vi "Main.vi"(11 "Module Admin":refnum<class "Delacor_lib_QMH_Module Admin.lvclass">) -> ()   [LabVIEW 2024, in "ProductControl.lvlib"]
doc: "This template is based off of the Queued Message Handler design pattern and the Queued Message Handler project template that ships with LabVIEW.\n\nThe main difference is that the queue is private to this module and communication between modules is performed via Broadcast and Request events.\n\nRequest events are wrapped in public API methods and are handled in the Event Handling Loop (EHL) of this VI. Any module can register for Broadcast events sent by this module. The EHL generates messages based on user interface actions.\n\nThe Message Handling Loop (MHL) processes messages generated by the EHL, or by other messages. The messages are string values, so new messages can be added easily to the Message Cases case structure in the MHL. Each message cluster can also provide an optional value for Message Data, which is a variant that can be converted to whatever message-specific data is required.\n_____\nBased on DQMH Dev Tools: Project Template 7.1.0.1503."
uses:
  ProductControl.lvlib
  <vilib>/Delacor/Delacor QMH/Libraries/Module Admin_class/Delacor_lib_QMH_Module Admin.lvclass
  Module Data--cluster.ctl
  <vilib>/Utility/miscctls.llb/LVFontTypeDef.ctl
  Stop Argument--cluster.ctl
  <vilib>/Delacor/Delacor QMH/Libraries/Message Queue_class/Delacor_lib_QMH_Message Queue.lvclass/Delacor_lib_QMH_Message Queue.ctl
  <vilib>/Delacor/Delacor QMH/Libraries/Module Admin_class/Delacor_lib_QMH_Module Admin.lvclass/Delacor_lib_QMH_Module Admin.ctl
  Draw FP in Subpanel Argument--cluster.ctl
  Remove From Subpanel Argument--cluster.ctl
  Cargar Invenario Argument--cluster.ctl
  <vilib>/Delacor/Delacor QMH/Libraries/Message Queue_class/Delacor_lib_QMH_Enqueue Message (Single).vi
  <vilib>/Delacor/Delacor QMH/Libraries/Module Admin_class/Delacor_lib_QMH_Get External Launch.vi
  <vilib>/Delacor/Delacor QMH/Libraries/Message Queue_class/Delacor_lib_QMH_Message Queue.lvclass
  <vilib>/PantherLAB/Message Module/Libraries/Message/PantherLAB_lib_Message.lvlib
  <vilib>/PantherLAB/Table Module/src/Libraries/Table/PantherLAB_lib_Table.lvlib
panel:
  out "error out":errorcluster
  out "Status":string
  in  "Comprar":bool
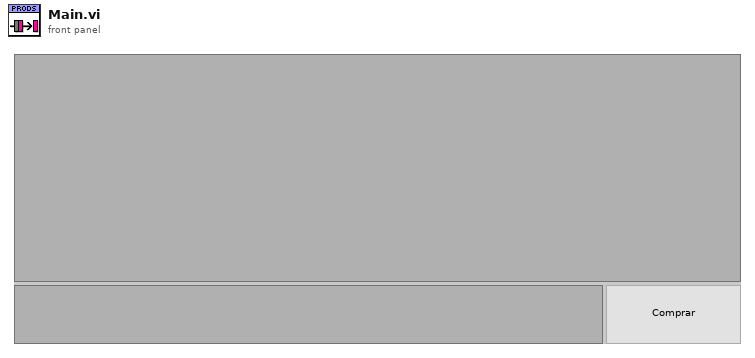
[diagram p1: front panel]
types:
  T1 = typedef "ProductControl.lvlib/Request Events--cluster.ctl" = cluster{"Stop Module":refnum<user-event>, "Show Panel":refnum<user-event>, "Hide Panel":refnum<user-event>, "Get Module Execution Status":refnum<user-event>, "Show Diagram":refnum<user-event>, "Draw FP in Subpanel":refnum<user-event>, "Remove From Subpanel":refnum<user-event>, "Private.Cargar Invenario":refnum<user-event>}
  T2 = typedef "PantherLAB_lib_Message.lvlib/Broadcast Events--cluster.ctl" = cluster{"Module Did Init":refnum<user-event>, "Status Updated":refnum<user-event>, "Error Reported":refnum<user-event>, "Module Did Stop":refnum<user-event>, "Update Module Execution Status":refnum<user-event>}
  T3 = typedef "PantherLAB_lib_Table.lvlib/Broadcast Events--cluster.ctl" = cluster{"Module Did Init":refnum<user-event>, "Status Updated":refnum<user-event>, "Error Reported":refnum<user-event>, "Module Did Stop":refnum<user-event>, "Update Module Execution Status":refnum<user-event>, "Selection Changed":refnum<user-event>}
  T4 = typedef "ProductControl.lvlib/Module Data--cluster.ctl" = cluster{"Status":string, "Sub Panel":refnum<vi>}
  T5 = typedef "LVFontTypeDef.ctl" = cluster{"Font Name":string, "Size":u16, "Bold":bool, "Italic":bool, "Underline":bool, "Strikeout":bool, "Color":u32}
  T6 = enum32{"invalid lock state", "Not Locked", "Locked (No Password)", "Password-protected"}
  T7 = typedef "ProductControl.lvlib/Stop Argument--cluster.ctl" = cluster{"Origin":string, "Exit via Stop Module Req?":bool, "Wait for Module to stop?":bool}
  T8 = typedef "ProductControl.lvlib/Draw FP in Subpanel Argument--cluster.ctl" = cluster{"Sub Panel":refnum<vi>}
  T9 = typedef "ProductControl.lvlib/Remove From Subpanel Argument--cluster.ctl" = cluster{"Boolean":bool}
  T10 = typedef "ProductControl.lvlib/Cargar Invenario Argument--cluster.ctl" = cluster{"Boolean":bool}
  T11 = enum32{"Invalid", "Standard", "Closed", "Hidden", "Minimized", "Maximized"}
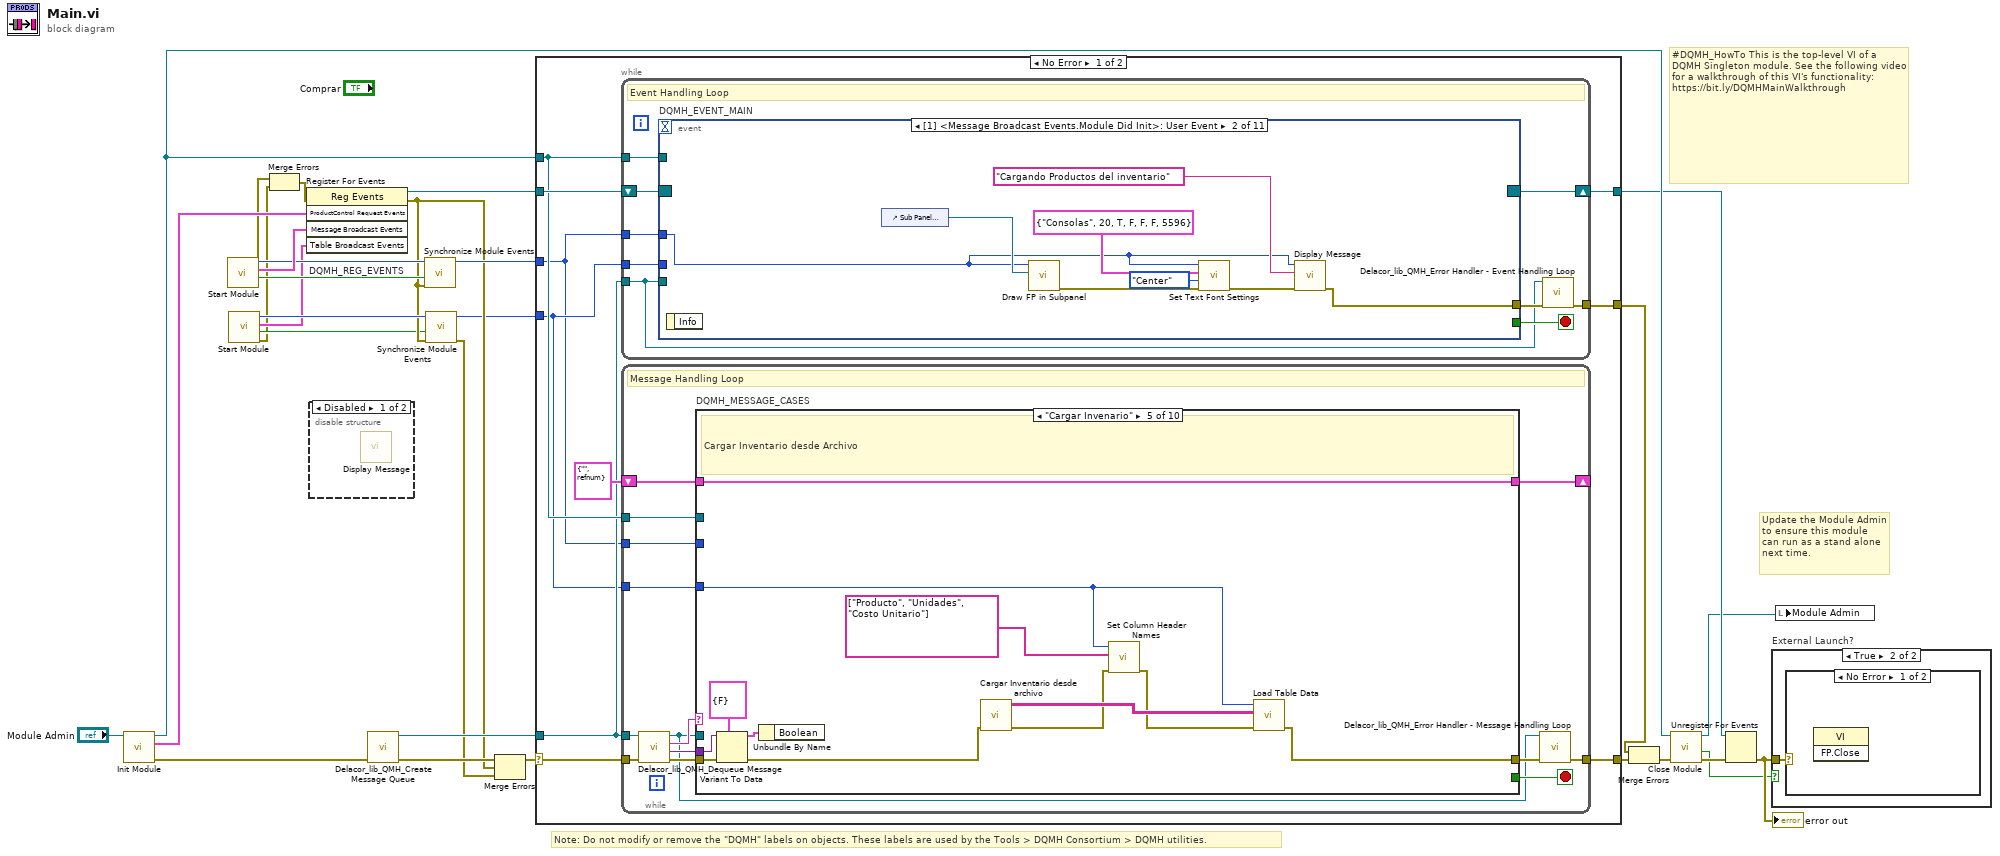
[diagram p0: block diagram]
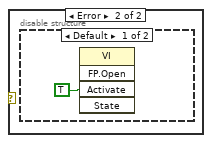
[diagram p4: hidden frame]
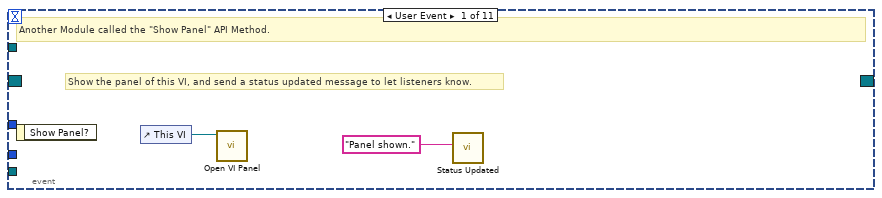
[diagram p6: hidden frame]
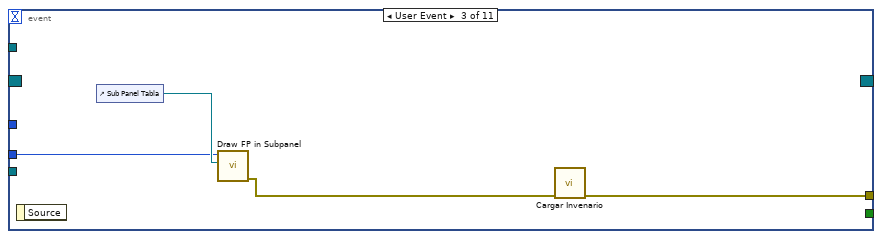
[diagram p7: hidden frame]
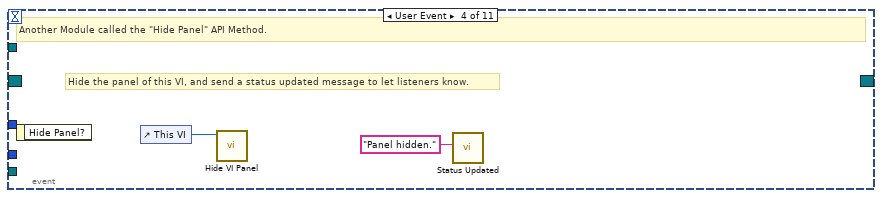
[diagram p8: hidden frame]
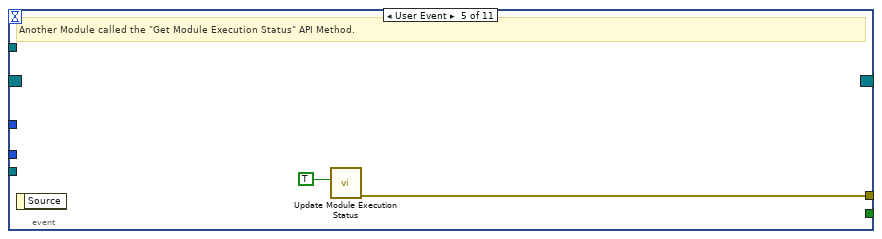
[diagram p9: hidden frame]
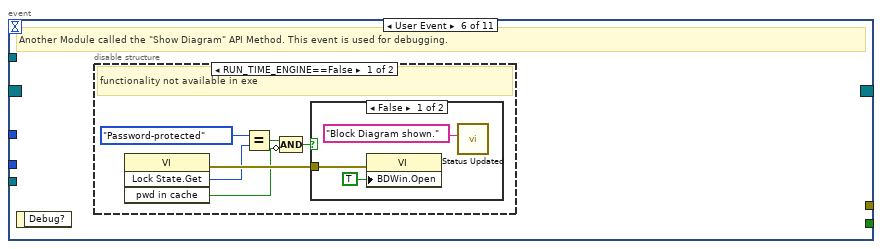
[diagram p10: hidden frame]
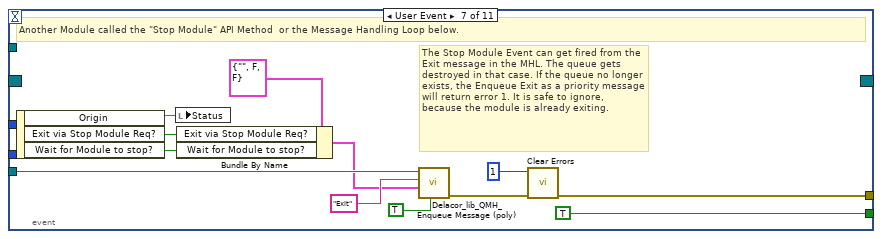
[diagram p13: hidden frame]
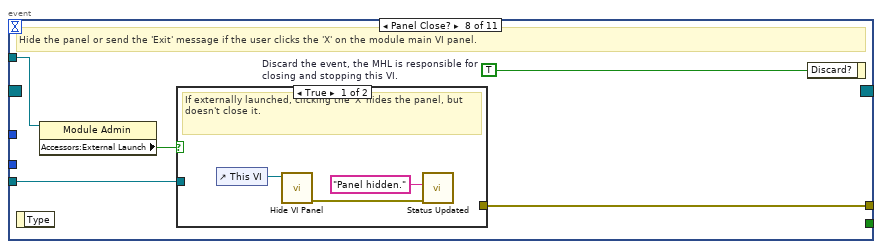
[diagram p14: hidden frame]
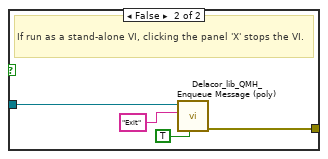
[diagram p15: hidden frame]
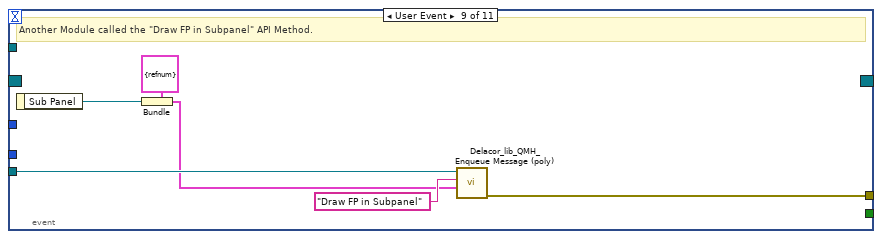
[diagram p16: hidden frame]
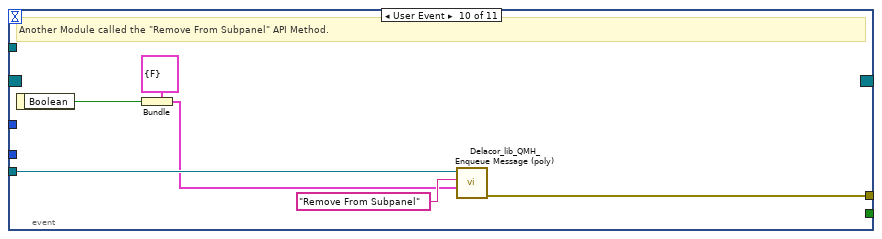
[diagram p17: hidden frame]
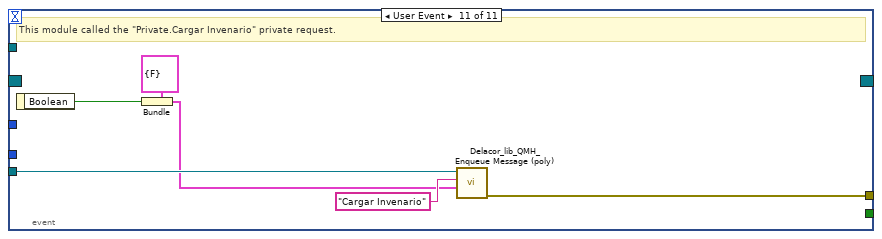
[diagram p18: hidden frame]
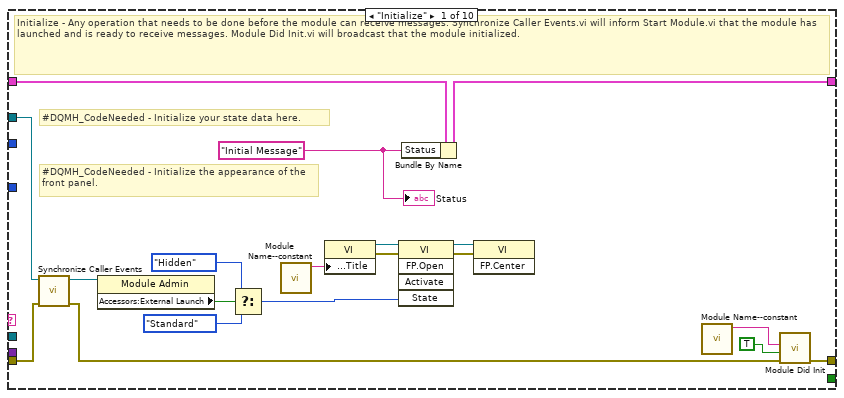
[diagram p19: hidden frame]
diagram:
  # "#DQMH_HowTo This is the top-level VI of a DQMH Singleton module. See the following video for a walkthrough of this VI's functionality: https://bit.ly/DQMHMainWalkthrough"
  # "Note: Do not modify or remove the \"DQMH\" labels on objects. These labels are used by the Tools > DQMH Consortium > DQMH utilities."
  # "Update the Module Admin to ensure this module can run as a stand alone next time."
  n1 = call "Init Module.vi"("Singleton Module Admin in"="Module Admin") -> ("error out"=w28:errorcluster, "ProductControl Request Events"=w18:T1, "Singleton Module Admin out"=w21:refnum<class "Delacor_lib_QMH_Module Admin.lvclass">)  [unwired: 8 in]
  n2 = call <vilib>:"Start Module.vi"() -> ("error out"=w9:errorcluster, "Wait for Event Sync?"=w12:bool, "Message Broadcast Events"=w11:T2, "Module ID"=w10:i32)  [unwired: 7 in, 1 out]
  n3 = call <vilib>:"Start Module.vi"() -> ("error out"=w2:errorcluster, "Wait for Event Sync?"=w4:bool, "Table Broadcast Events"=w5:T3, "Module ID"=w8:i32)  [unwired: 7 in, 1 out]
  n4 = Merge Errors(w9, w2) -> (w3:errorcluster)
  n5 = register-events "DQMH_REG_EVENTS"(error in=w3, w18, w11, w5) -> (reference out=w19:refnum<event-registration>, error out=w7:errorcluster)  [unwired: 1 in]
  n6 = disable-structure shown="Disabled" {
    frame Disabled {
      n7 = call <vilib>:"Display Message.vi"() -> ()  [unwired: 11 in, 1 out]
    }
    frame Enabled {
    }
  }
  n8 = call <vilib>:"Delacor_lib_QMH_Create Message Queue.vi"("error in"=w28) -> ("error out"=w23:errorcluster, "Message Queue"=w17:refnum<class "Delacor_lib_QMH_Message Queue.lvclass">)  [unwired: 9 in]
  n9 = call <vilib>:"Synchronize Module Events.vi"("error in"=w7, "Wait for Event Sync?"=w12, "Module ID in"=w10) -> ("Module ID out"=w13:i32)  [unwired: 7 in, 1 out]
  n10 = call <vilib>:"Synchronize Module Events.vi"("error in"=w7, "Wait for Event Sync?"=w4, "Module ID in"=w8) -> ("error out"=w6:errorcluster, "Module ID out"=w1:i32)  [unwired: 7 in]
  n11 = Merge Errors(w23, w7, w6) -> (w22:errorcluster)
  n12 = case shown="No Error" w22 {
    selector: w22 -> [w37 w262]
    tunnel: [w39 w261] -> w29
    tunnel: [w36 w260] -> w20
    tunnel: w19 -> [w34 w260]
    tunnel: w17 -> [w32 w256]
    tunnel: [w38 _] -> w26
    tunnel: w21 -> [w33 w257]
    tunnel: w13 -> [w30 w254]
    tunnel: w1 -> [w31 _]
    frame No Error {
      n13 = while {
        tunnel: w32 -> [w42]
        shift-right: [w45] -> w36
        shift-left: w34 -> [w46]
        tunnel: [w47] -> w38
        tunnel: w33 -> [w43]
        tunnel: w31 -> [w41]
        tunnel: w30 -> [w40]
        stop <- w44 stop-if-true
        # "Event Handling Loop"
        n14 = event "DQMH_EVENT_MAIN" shown="[1] <Message Broadcast Events.Module Did Init>: User Event" {
          selector: w46 -> [_ _ _ _ _ _ _ _ _ _ _]
          dyn-events: [_ _ _ _ _ _ _ _ _ _ _] -> w45
          timeout: _ -> [_ _ _ _ _ _ _ _ _ _ _]
          tunnel: [_ _ _ _ _ _ TRUE ("Discard?") _ _ _ _] -> w44
          tunnel: w42 -> [_ _ _ _ _ _ w83 w90 w104 w110 w117]
          tunnel: [_ w55 w60 _ w66 _ w86 w92 w105 w111 w112] -> w48
          tunnel: w43 -> [_ _ _ _ _ _ _ w89 _ _ _]
          tunnel: w41 -> [_ _ w59 _ _ _ _ _ _ _ _]
          tunnel: w40 -> [_ w51 _ _ _ _ _ _ _ _ _]
          event User Event {
            # "Show the panel of this VI, and send a status updated message to let listeners know."
            # "Another Module called the \"Show Panel\" API Method."
            n15 = event-data() -> ()  [unwired: 1 in, 1 out]
            n16 = control-ref of="This VI"() -> (w50:refnum<vi>)
            n17 = call "Open VI Panel.vi"("VI"=w50) -> ()  [unwired: 10 in, 1 out]
            n18 = call "Status Updated.vi"("Status"="Panel shown." ("format string")) -> ()  [unwired: 10 in, 1 out]
          }
          event User Event {
            n19 = event-data() -> ()  [unwired: 1 in, 1 out]
            n20 = control-ref of="Sub Panel Mensajes"() -> (w58:refnum<vi>)
            n21 = call <vilib>:"Draw FP in Subpanel.vi"("Sub Panel"=w58, "Module ID"=w51) -> ("error out"=w57:errorcluster)  [unwired: 9 in]
            n22 = call <vilib>:"Set Text Font Settings.vi"("error in"=w57, "Text.Justification"=enum16{"Left", "Center", "Right"}."Center", "Font"=T5 {"Font Name"="Consolas", "Size"=20, "Bold"=TRUE, "Italic"=FALSE, "Underline"=FALSE, "Strikeout"=FALSE, "Color"=5596}, "Module ID"=w51) -> ("error out"=w56:errorcluster)  [unwired: 7 in]
            n23 = call <vilib>:"Display Message.vi"("error in"=w56, "Message"="Cargando Productos del inventario", "Module ID"=w51) -> ("error out"=w55:errorcluster)  [unwired: 8 in]
          }
          event User Event {
            n24 = event-data() -> ()  [unwired: 1 in, 1 out]
            n25 = control-ref of="Sub Panel Tabla"() -> (w62:refnum<vi>)
            n26 = call <vilib>:"Draw FP in Subpanel.vi"("Sub Panel"=w62, "Module ID"=w59) -> ("error out"=w61:errorcluster)  [unwired: 9 in]
            n27 = call "Cargar Invenario.vi"("error in"=w61) -> ("error out"=w60:errorcluster)  [unwired: 10 in]
          }
          event User Event {
            # "Hide the panel of this VI, and send a status updated message to let listeners know."
            # "Another Module called the \"Hide Panel\" API Method."
            n28 = event-data() -> ()  [unwired: 1 in, 1 out]
            n29 = control-ref of="This VI"() -> (w64:refnum<vi>)
            n30 = call "Hide VI Panel.vi"("VI"=w64) -> ()  [unwired: 10 in, 1 out]
            n31 = call "Status Updated.vi"("Status"="Panel hidden." ("format string")) -> ()  [unwired: 10 in, 1 out]
          }
          event User Event {
            # "Another Module called the \"Get Module Execution Status\" API Method."
            n32 = event-data() -> ()  [unwired: 1 in, 1 out]
            n33 = call "Update Module Execution Status.vi"("Running?"=TRUE) -> ("error out"=w66:errorcluster)  [unwired: 10 in]
          }
          event User Event {
            # "Another Module called the \"Show Diagram\" API Method. This event is used for debugging."
            n34 = event-data() -> ()  [unwired: 1 in, 1 out]
            n35 = disable-structure shown="RUN_TIME_ENGINE==False" {
              frame condition #0 (active) {
                # "functionality not available in exe"
                n36 = invoke on="Invoke Node" class="VI" method="Lock State.Get"() -> (error out=w72:errorcluster, "Get Lock State"=w71:T6, "pwd in cache"=w68:bool)  [unwired: 4 in, 1 out]
                n37 = Equal?(x=T6."Password-protected", y=w71) -> (x = y?=w69:bool)
                n38 = Compound Arithmetic op=AND(w69, invert w68) -> (w67:bool)
                n39 = case shown="False" w67 {
                  tunnel: w72 -> [w75 _]
                  frame False {
                    n40 = property on="Property Node" class="VI"(error in=w75, "BDWin.Open"=TRUE ("Block Diagram Window:Open")) -> ()  [unwired: 1 in, 2 out]
                    n41 = call "Status Updated.vi"("Status"="Block Diagram shown." ("format string")) -> ()  [unwired: 10 in, 1 out]
                  }
                  frame True {
                    # "Password-protected VI, and the password is not in the cache. Do not show the diagram."
                  }
                }
              }
              frame condition #1 {
              }
            }
          }
          event User Event {
            # "The Stop Module Event can get fired from the Exit message in the MHL. The queue gets destroyed in that case. If the queue no longer exists, the Enqueue Exit as a priority message will return error 1. It is safe to ignore, because the module is already exiting."
            # "Another Module called the \"Stop Module\" API Method  or the Message Handling Loop below."
            n42 = event-data() -> ("Origin"=w82:string, "Exit via Stop Module Req?"=w78:bool, "Wait for Module to stop?"=w77:bool)  [unwired: 1 in]
            n43 = local write "Status"(w82) -> ()
            n44 = Bundle By Name(cluster=T7 {"Origin"="", "Exit via Stop Module Req?"=FALSE, "Wait for Module to stop?"=FALSE} ("Stop Argument"), "Exit via Stop Module Req?"=w78, "Wait for Module to stop?"=w77) -> (w76:T7)
            n45 = call-poly <vilib>:"Delacor_lib_QMH_Enqueue Message (poly).vi"("Priority Message? (F)"=TRUE, "Message Data"=w76, "Message"="Exit", "Message Queue in"=w83) -> ("error out"=w87:errorcluster)  [unwired: 6 in, 1 out]
            n46 = call <vilib>:"Clear Errors.vi"("error in (no error)"=w87, "specific error code to clear (0: all)"=1) -> ("error out"=w86:errorcluster)  [unwired: 4 in, 1 out]
          }
          event Panel Close? {
            w91 = TRUE  # Discard the event, the MHL is responsible for closing and stopping this VI.
            # "Hide the panel or send the 'Exit' message if the user clicks the 'X' on the module main VI panel."
            n47 = event-data() -> ()  [unwired: 1 in, 1 out]
            n48 = property on="Property Node" class="Module Admin"(reference=w89) -> ("Accessors:External Launch"=w88:bool)  [unwired: 1 in, 2 out]
            n49 = case shown="True" w88 {
              tunnel: w90 -> [_ w98]
              tunnel: [_ w99] -> w92
              frame True {
                # "If externally launched, clicking the 'X' hides the panel, but doesn't close it."
                n50 = control-ref of="This VI"() -> (w94:refnum<vi>)
                n51 = call "Hide VI Panel.vi"("VI"=w94) -> ("error out"=w95:errorcluster)  [unwired: 10 in]
                n52 = call "Status Updated.vi"("error in"=w95, "Status"="Panel hidden." ("format string")) -> ()  [unwired: 9 in, 1 out]
              }
              frame False {
                # "If run as a stand-alone VI, clicking the panel 'X' stops the VI."
                n53 = call-poly <vilib>:"Delacor_lib_QMH_Enqueue Message (poly).vi"("Priority Message? (F)"=TRUE, "Message"="Exit", "Message Queue in"=w98) -> ("error out"=w99:errorcluster)  [unwired: 7 in, 1 out]
              }
            }
            n54 = event-data ("Event Filter Node")("Discard?"=w91) -> ()  [unwired: 1 in, 1 out]
          }
          event User Event {
            # "Another Module called the \"Draw FP in Subpanel\" API Method."
            n55 = event-data() -> ("Sub Panel"=w100:refnum<vi>)  [unwired: 1 in]
            n56 = Bundle(cluster=T8 {"Sub Panel"=refnum} ("Draw FP in Subpanel Argument"), "Sub Panel"=w100) -> (w101:T8)
            n57 = call-poly <vilib>:"Delacor_lib_QMH_Enqueue Message (poly).vi"("Message Data"=w101, "Message"="Draw FP in Subpanel", "Message Queue in"=w104) -> ("error out"=w105:errorcluster)  [unwired: 7 in, 1 out]
          }
          event User Event {
            # "Another Module called the \"Remove From Subpanel\" API Method."
            n58 = event-data() -> ("Boolean"=w106:bool)  [unwired: 1 in]
            n59 = Bundle(cluster=T9 {"Boolean"=FALSE} ("Remove From Subpanel Argument"), "Boolean"=w106) -> (w107:T9)
            n60 = call-poly <vilib>:"Delacor_lib_QMH_Enqueue Message (poly).vi"("Message Data"=w107, "Message"="Remove From Subpanel", "Message Queue in"=w110) -> ("error out"=w111:errorcluster)  [unwired: 7 in, 1 out]
          }
          event User Event {
            # "This module called the \"Private.Cargar Invenario\" private request."
            n61 = event-data() -> ("Boolean"=w113:bool)  [unwired: 1 in]
            n62 = Bundle(cluster=T10 {"Boolean"=FALSE} ("Cargar Invenario Argument"), "Boolean"=w113) -> (w114:T10)
            n63 = call-poly <vilib>:"Delacor_lib_QMH_Enqueue Message (poly).vi"("Message Data"=w114, "Message"="Cargar Invenario", "Message Queue in"=w117) -> ("error out"=w112:errorcluster)  [unwired: 7 in, 1 out]
          }
        }
        n64 = call-dynamic "Delacor_lib_QMH_Error Handler - Event Handling Loop.vi"("error in"=w48, "Message Queue in"=w42) -> ("dup error in"=w47:errorcluster)  [unwired: 8 in, 1 out]
      }
      n65 = while {
        tunnel: w32 -> [w120]
        shift-right: [w126] -> _
        shift-left: T4 {"Status"="", "Sub Panel"=refnum} ("Data Cluster") -> [w127]
        tunnel: w37 -> [w131]
        tunnel: [w129] -> w39
        tunnel: w33 -> [w122]
        tunnel: w30 -> [w119]
        tunnel: w31 -> [w118]
        stop <- w125 stop-if-true
        # "Message Handling Loop"
        n66 = call-dynamic "Delacor_lib_QMH_Dequeue Message.vi"("error in"=w131, "Message Queue in"=w120) -> ("error out"=w130:errorcluster, "Message Data"=w123:variant, "Message"=w124:string, "Message Queue out"=w121:refnum<class "Delacor_lib_QMH_Message Queue.lvclass">)  [unwired: 6 in]
        n67 = case "DQMH_MESSAGE_CASES" shown="\"Cargar Invenario\"" w124 {
          selector: w124 -> [_ _ _ _ _ _ _ _ _ w249]
          tunnel: w121 -> [_ _ _ _ _ _ _ w212 w237 _]
          tunnel: w130 -> [w148 w152 w168 w186 w204 w207 w209 w220 w243 w252]
          tunnel: [w146 w152 w167 w184 w199 w206 w209 w216 w238 w253] -> w128
          tunnel: w127 -> [w137 w151 w163 w180 w203 w205 w208 w214 w229 w250]
          tunnel: [w136 w151 w159 w177 w203 w205 w208 w214 w229 w250] -> w126
          tunnel: [_ _ _ _ _ _ _ _ w236 _] -> w125
          tunnel: w123 -> [_ _ w162 w183 w202 _ _ w213 w235 _]
          tunnel: w122 -> [w138 _ _ _ _ _ _ w211 w230 _]
          tunnel: w119 -> [_ _ _ _ _ _ _ _ w227 _]
          tunnel: w118 -> [_ _ _ _ w194 _ _ _ _ _]
          frame "Initialize" {
            w132 = "Initial Message" ("Initial Message")
            # "#DQMH_CodeNeeded - Initialize the appearance of the front panel."
            # "#DQMH_CodeNeeded - Initialize your state data here."
            # "Initialize - Any operation that needs to be done before the module can receive messages. Synchronize Caller Events.vi will inform Start Module.vi that the module has launched and is ready to receive messages. Module Did Init.vi will broadcast that the module initialized."
            n68 = call "Synchronize Caller Events.vi"("error in"=w148, "Singleton Module Admin in"=w138) -> ("error out"=w147:errorcluster, "Singleton Module Admin out"=w133:refnum<class "Delacor_lib_QMH_Module Admin.lvclass">)  [unwired: 8 in]
            n69 = property on="Property Node" class="Module Admin"(reference=w133) -> ("Accessors:External Launch"=w142:bool)  [unwired: 1 in, 2 out]
            n70 = Select(t=T11."Hidden" ("State"), s=w142, f=T11."Standard" ("State")) -> (s? t:f=w139:T11)
            n71 = call "Module Name--constant.vi"() -> ("Module Name"=w145:string)  [unwired: 11 in]
            n72 = property on="Property Node" class="VI"("Front Panel.Title"=w145) -> (reference out=w144:refnum<vi>, error out=w150:errorcluster)  [unwired: 2 in]
            n73 = invoke on="Invoke Node" class="VI" method="FP.Open"(reference=w144, error in=w150, "State"=w139) -> (reference out=w143:refnum<vi>, error out=w149:errorcluster)  [unwired: 2 in, 3 out]
            n74 = Bundle By Name(cluster=w137, "Status"=w132) -> (w136:T4)
            n75 = invoke on="Invoke Node" class="VI" method="FP.Center"(reference=w143, error in=w149) -> ()  [unwired: 1 in, 3 out]
            n76 = call "Module Name--constant.vi"() -> ("Module Name"=w134:string)  [unwired: 11 in]
            n77 = call "Module Did Init.vi"("error in"=w147, "Initialized?"=TRUE, "Origin"=w134) -> ("error out"=w146:errorcluster)  [unwired: 8 in]
            "Status" <- w132
          }
          frame "---Module Specific---" {
            # "Separator -- The following cases handle messages specific to this Module."
          }
          frame "Draw FP in Subpanel" {
            # "Draw FP in Subpanel"
            n78 = Variant To Data(error in=w168, type=T8 {"Sub Panel"=refnum} ("Draw FP in Subpanel Argument"), Variant=w162) -> (data=w160:T8, error out=w166:errorcluster)
            n79 = Unbundle By Name(w160) -> ("Sub Panel"=w158:refnum<vi>)
            n80 = control-ref of="This VI"() -> (w155:refnum<vi>)
            n81 = property class="VI"(reference=w155, error in=w166) -> (reference out=w154:refnum<vi>, error out=w164:errorcluster, "FP.State"=w153:T11)
            n82 = case shown="\"Closed\"" w153 {
              tunnel: [w169 w172] -> w156
              tunnel: [w170 w174] -> w165
              tunnel: w164 -> [w170 w173]
              tunnel: w154 -> [w169 w171]
              frame "Closed" {
              }
              frame "Standard", Default {
                n83 = invoke class="VI" method="FP.Close"(reference=w171, error in=w173) -> (reference out=w172:refnum<vi>, error out=w174:errorcluster)  [unwired: 1 in, 1 out]
              }
            }
            n84 = invoke class="SubPnl" method="Insert VI"(reference=w158, error in=w165, "VI Ref"=w156) -> (reference out=w157:refnum<vi>, error out=w167:errorcluster)  [unwired: 1 in, 2 out]
            n85 = Bundle By Name(cluster=w163, "Sub Panel"=w157) -> (w159:T4)
          }
          frame "Remove From Subpanel" {
            # "Remove From Subpanel"
            n86 = Variant To Data(error in=w186, type=T9 {"Boolean"=FALSE} ("Remove From Subpanel Argument"), Variant=w183) -> (data=w181:T9, error out=w185:errorcluster)
            n87 = Unbundle By Name(w181) -> ()  [unwired: 1 out]
            n88 = Unbundle By Name(w180) -> ("Sub Panel"=w179:refnum<vi>)
            n89 = Not A Number/Path/Refnum?(number/path/refnum=w179) -> (NaN/Path/Refnum?=w178:bool)
            n90 = case shown="True" w178 {
              tunnel: w185 -> [w190 w192]
              tunnel: [w189 w192] -> w184
              tunnel: w179 -> [w188 _]
              tunnel: ["Module Removed from Subpanel" "This module has not been inserted into the subpanel"] -> w175
              frame False {
                n91 = invoke class="SubPnl" method="Remove VI"(reference=w188, error in=w190) -> (error out=w189:errorcluster)  [unwired: 1 in, 2 out]
              }
              frame True {
              }
            }
            n92 = Bundle By Name(cluster=w180, "Sub Panel"=refnum<vi> refnum) -> (w177:T4)
            n93 = call "Status Updated.vi"("Status"=w175) -> ()  [unwired: 10 in, 1 out]
          }
          frame "Cargar Invenario" {
            # "Cargar Inventario desde Archivo"
            n94 = Variant To Data(error in=w204, type=T10 {"Boolean"=FALSE} ("Cargar Invenario Argument"), Variant=w202) -> (data=w200:T10, error out=w198:errorcluster)
            n95 = Unbundle By Name(w200) -> ()  [unwired: 1 out]
            n96 = call "Cargar Inventario desde archivo.vi"("error in"=w198) -> ("error out"=w196:errorcluster, "Productos"=w197:string[][])  [unwired: 9 in]
            n97 = call <vilib>:"Set Column Header Names.vi"("error in"=w196, "Column Names"=string[] ["Producto", "Unidades", "Costo Unitario"], "Module ID"=w194) -> ("error out"=w195:errorcluster)  [unwired: 8 in]
            n98 = call <vilib>:"Load Table Data.vi"("error in"=w195, "Table Data"=w197, "Module ID"=w194) -> ("error out"=w199:errorcluster)  [unwired: 8 in]
          }
          frame "---Copy This Frame---" {
            # "Duplicate this frame when creating new messages.  Change this comment in the duplicated frame to describe this message."
            n99 = Merge Errors(w207) -> (w206:errorcluster)
          }
          frame "---Exit and Error Handling---" {
            # "Separator - The following cases handle errors and exit messages."
          }
          frame "Error" {
            # "#DQMH_CodeRecommended - If the module is running in standalone mode (External Launch = FALSE), this code will pop up an error dialog and call the 'Exit' message if an error occurs. Add more fine-grained error management here."
            # "Error - Check the error message data and respond accordingly. This message is sent by the \"Error Handler\" VIs at the end of each loop in this application."
            n100 = property on="Property Node" class="Module Admin"(reference=w211) -> ("Accessors:External Launch"=w210:bool)  [unwired: 1 in, 2 out]
            n101 = Variant To Data(error in=w220, type=errorcluster {"status"=FALSE, "code"=0, "source"=""} ("error constant"), Variant=w213) -> (data=w215:errorcluster, error out=w218:errorcluster)
            n102 = local write "error out"(w215) -> ()
            n103 = call "Error Reported.vi"("Error"=w215) -> ()  [unwired: 10 in, 1 out]
            n104 = case shown="False" w210 {
              tunnel: [w225 _] -> w217
              tunnel: w212 -> [w223 _]
              tunnel: w215 -> [w224 _]
              frame False {
                n105 = disable-structure shown="Default" {
                  disable-tunnel: w224 -> [w226 _]
                  frame condition #0 (active) {
                    # "If the module is running standalone, then pop up an error dialog and call the \"Exit\" message."
                    n106 = call <vilib>:"Simple Error Handler.vi"("error in (no error)"=w226) -> ()  [unwired: 4 in, 5 out]
                  }
                  frame condition #1 {
                    # "To prevent the Simple Error Handler VI from being loaded (e.g. when deploying to a Real-Time target), add the Conditional Disable Symbol \"DQMH_Disable_SEH\" to your project and set it to TRUE."
                  }
                }
                n107 = call-poly <vilib>:"Delacor_lib_QMH_Enqueue Message (poly).vi"("Priority Message? (F)"=TRUE, "Message"="Exit", "Message Queue in"=w223) -> ("error out"=w225:errorcluster)  [unwired: 7 in, 1 out]
              }
              frame True {
                # "If the module was launched externally, calling the Error Reported broadcast VI is the only action performed by the \"Error\" message. The module's caller can then process the error appropriately."
              }
            }
            n108 = Merge Errors(w218, w217) -> (w216:errorcluster)
          }
          frame "Exit" {
            w234 = 91  # 91: not all Exit messages will have an argument
            w236 = TRUE  # Stop the VI
            # "Release the message queue reference"
            # "#DQMH_CodeNeeded - Add any required cleanup code here."
            # "Exit - Exit the application."
            n109 = Variant To Data(error in=w243, type=T7 {"Origin"="", "Exit via Stop Module Req?"=FALSE, "Wait for Module to stop?"=FALSE} ("Stop Argument"), Variant=w235) -> (data=w232:T7, error out=w240:errorcluster)
            n110 = call <vilib>:"Clear Errors.vi"("error in (no error)"=w240, "specific error code to clear (0: all)"=w234) -> ("error out"=w242:errorcluster)  [unwired: 4 in, 1 out]
            n111 = control-ref of="This VI"() -> (w231:refnum<vi>)
            n112 = call-dynamic "Delacor_lib_QMH_Release Message Queue.vi"("error in"=w242, "Message Queue"=w237) -> ("error out"=w241:errorcluster)  [unwired: 9 in]
            n113 = call "Handle Exit.vi"("Stop Argument"=w232, "Admin in"=w230, "VI reference"=w231) -> ("error out"=w239:errorcluster)  [unwired: 7 in, 1 out]
            n114 = Merge Errors(w241, w239) -> (w238:errorcluster)
            n115 = Unbundle By Name(w229) -> ("Sub Panel"=w228:refnum<vi>)
            n116 = call "Error Reported.vi"("Error"=w238) -> ()  [unwired: 10 in, 1 out]
            n117 = invoke class="SubPnl" method="Remove VI"(reference=w228) -> ()  [unwired: 2 in, 3 out]
            n118 = call <vilib>:"Stop Module.vi"("Module ID"=w227) -> ()  [unwired: 10 in, 1 out]
          }
          frame Default {
            # "'Default' case only runs if there is a message that isn't defined in any of the other cases.  Output a programming error."
            n119 = call "Module Name--constant.vi"() -> ("Module Name"=w248:string)  [unwired: 11 in]
            n120 = Format Into String(format string="The invalid message string \"%s\" was received in the Message Handling Loop for module \"%s\".", w249, w248) -> (resulting string=w244:string)  [unwired: 2 in, 1 out]
            n121 = call <vilib>:"Error Cluster From Error Code.vi"("show call chain? (False)"=TRUE, "error message (\"\")"=w244, "error code (0)"=1) -> ("error out"=w251:errorcluster)  [unwired: 6 in]
            n122 = Merge Errors(w252, w251) -> (w253:errorcluster)
          }
        }
        n123 = call-dynamic "Delacor_lib_QMH_Error Handler - Message Handling Loop.vi"("error in"=w128, "Message Queue in"=w121) -> ("dup error in"=w129:errorcluster)  [unwired: 8 in, 1 out]
      }
    }
    frame Error {
      # "Synchronize Caller Events.vi will inform Start Module.vi that the module has launched and will let the code calling Start Module.vi register for broadcasts and would permit the caller receive the broadcast that an error occurred at launch time."
      n124 = call-dynamic "Delacor_lib_QMH_Release Message Queue.vi"("error in"=w262, "Message Queue"=w256) -> ("error out"=w261:errorcluster)  [unwired: 9 in]
      n125 = call "Synchronize Caller Events.vi"("Singleton Module Admin in"=w257) -> ("error out"=w263:errorcluster)  [unwired: 9 in, 1 out]
      n126 = call "Module Name--constant.vi"() -> ("Module Name"=w259:string)  [unwired: 11 in]
      n127 = Format Into String(format string="An error occurred during initialization. %s is no longer running.", w259) -> (resulting string=w255:string)  [unwired: 2 in, 1 out]
      n128 = Merge Errors(w261, w263) -> (w264:errorcluster)
      n129 = call "Error Reported.vi"("Additional Information"=w255, "Error"=w264) -> ()  [unwired: 9 in, 1 out]
      n130 = call <vilib>:"Stop Module.vi"("Origin"=w255, "Module ID"=w254) -> ()  [unwired: 9 in, 1 out]
    }
  }
  n131 = Merge Errors(w26, w29) -> (w25:errorcluster)
  n132 = call "Close Module.vi"("error in"=w25, "Module Admin in"=w21) -> ("error out"=w27:errorcluster, "External Launch"=w14:bool, "Module Admin out"=w15:refnum<class "Delacor_lib_QMH_Module Admin.lvclass">)  [unwired: 7 in]
  n133 = Unregister For Events(event registration refnum=w20, error in=w27) -> (error out=w24:errorcluster)
  "error out" <- w24
  n134 = case "External Launch?" shown="True" w14 {
    tunnel: w24 -> [_ w265]
    frame False {
    }
    frame True {
      n135 = case shown="No Error" w265 {
        frame No Error {
          n136 = invoke on="Invoke Node" class="VI" method="FP.Close"() -> ()  [unwired: 3 in, 3 out]
        }
        frame Error {
          n137 = disable-structure shown="Default" {
            frame condition #0 (active) {
              n138 = invoke class="VI" method="FP.Open"("Activate"=TRUE ("Activate?")) -> ()  [unwired: 4 in, 5 out]
            }
            frame condition #1 {
              # "Don't show panel on error if running inside a built EXE."
            }
          }
        }
      }
    }
  }
  n139 = local write "Module Admin"(w15) -> ()
